vi "Release SequenceFile.vi"(8 "error in (no error)":errorcluster, 10 "SequenceFile":refnum<k7>, 11 "Engine in":refnum<class "Engine.lvclass">) -> (0 "error out":errorcluster, 3 "Engine out":refnum<class "Engine.lvclass">)   [LabVIEW 2020, in "TSnax.lvlib" / "Engine.lvclass"]
uses:
  Engine.lvclass
  Engine.lvclass/Engine.ctl
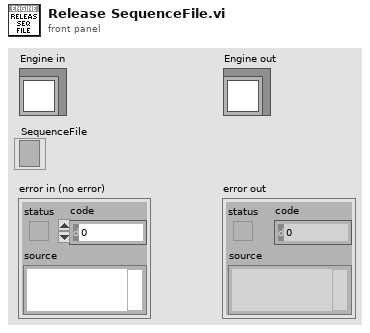
[diagram p1: front panel]
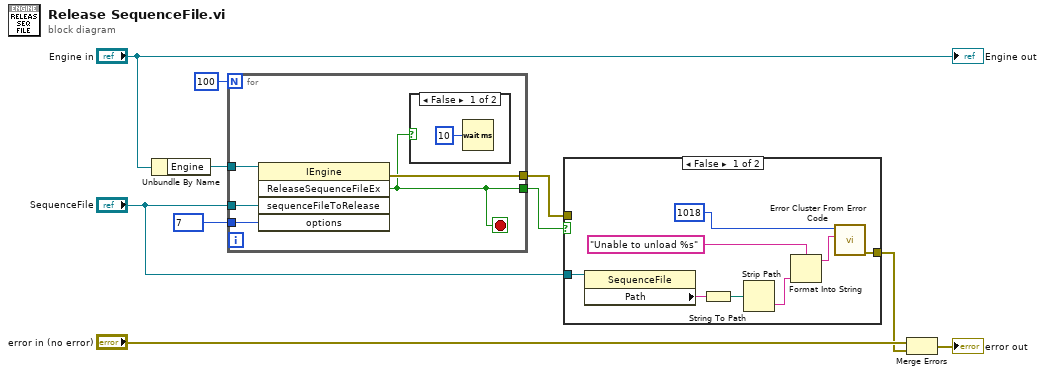
[diagram p0: block diagram]
diagram:
  n1 = Unbundle By Name("Engine in") -> ("Engine"=w7:refnum<k7>)
  n2 = for {
    N: 100 -> [_]
    tunnel: w7 -> [w15]
    tunnel: "SequenceFile" -> [w14]
    tunnel: 7 ("options") -> [w13]
    tunnel: [w11] -> w5
    tunnel: [w12] -> w4
    stop <- w11 stop-if-true
    n3 = invoke class="IEngine" method="ReleaseSequenceFileEx"(reference=w15, "sequenceFileToRelease"=w14, "options"=w13) -> (error out=w12:errorcluster, "ReleaseSequenceFileEx"=w11:bool)  [unwired: 2 in, 3 out]
    n4 = case shown="False" w11 {
      frame False {
        n5 = Wait (ms)(milliseconds to wait=u32 10) -> ()  [unwired: 1 out]
      }
      frame True {
      }
    }
  }
  n6 = case shown="False" w5 {
    tunnel: w4 -> [_ w25]
    tunnel: [w23 w25] -> w1
    tunnel: "SequenceFile" -> [w22 _]
    frame False {
      n7 = property class="SequenceFile"(reference=w22) -> ("Path"=w21:string)  [unwired: 1 in, 2 out]
      n8 = String To Path(string=w21) -> (path=w20:path)
      n9 = Strip Path(path=w20) -> (name=w18:string)  [unwired: 1 out]
      n10 = Format Into String(format string="Unable to unload %s" ("error message (\"\")"), w18) -> (resulting string=w17:string)  [unwired: 2 in, 1 out]
      n11 = call <vilib>:"Error Cluster From Error Code.vi"("error message (\"\")"=w17, "error code (0)"=1018) -> ("error out"=w23:errorcluster)  [unwired: 7 in]
    }
    frame True {
    }
  }
  n12 = Merge Errors("error in (no error)", w1) -> (→"error out":errorcluster)
  "Engine out" <- "Engine in"
